vi "Write AO_index.vi"(8 "error in (no error)":errorcluster, 10 "AO_index":u16, 11 "bronkhorst_reg in":refnum<class "bronkhorst_reg.lvclass">) -> (0 "error out":errorcluster, 3 "bronkhorst_reg out":refnum<class "bronkhorst_reg.lvclass">)   [LabVIEW 2019, in "bronkhorst_reg.lvclass"]
uses:
  bronkhorst_reg.lvclass
  bronkhorst_reg.lvclass/bronkhorst_reg.ctl
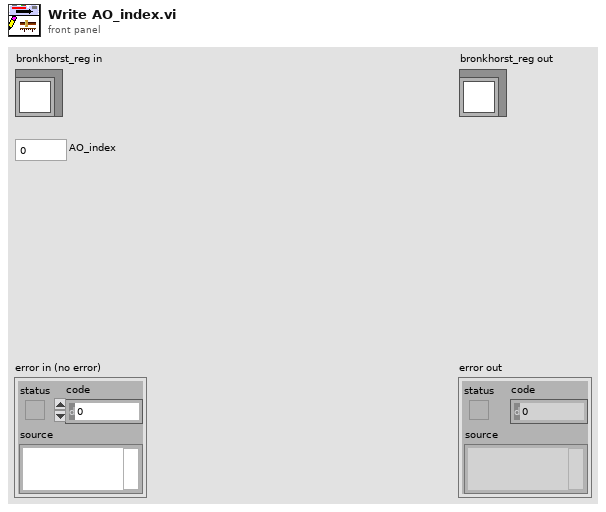
[diagram p1: front panel]
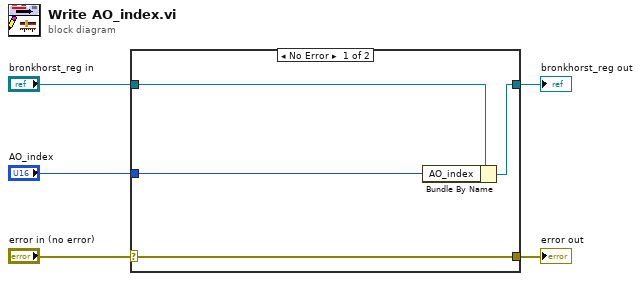
[diagram p0: block diagram]
diagram:
  n1 = case shown="No Error" "error in (no error)" {
    selector: "error in (no error)" -> [w9 w10]
    tunnel: [w9 w10] -> w4
    tunnel: [w7 w11] -> w2
    tunnel: "bronkhorst_reg in" -> [w8 w11]
    tunnel: "AO_index" -> [w6 _]
    frame No Error {
      n2 = Bundle By Name(cluster=w8, "AO_index"=w6) -> (w7:refnum<class "bronkhorst_reg.lvclass">)
    }
    frame Error {
    }
  }
  "error out" <- w4
  "bronkhorst_reg out" <- w2
